vi "Handle Error.vi"(8 "error in (no error)":errorcluster, 11 "ModelLogsAndClearsErrors in":refnum<class "ModelLogsAndClearsErrors.lvclass">) -> (0 "error out":errorcluster, 2 "stop actor?":bool=TRUE, 3 "ModelLogsAndClearsErrors out":refnum<class "ModelLogsAndClearsErrors.lvclass">)   [LabVIEW 2020, in "ModelLogsAndClearsErrors.lvclass"]
doc: "(<B>Filename</B>: Actor Framework.lvlib:Actor.lvclass:Handle Error.vi)\n\nDefines how the actor handles an error that occurred while processing a message. By default, this method does nothing except stop the actor."
uses:
  ModelLogsAndClearsErrors.lvclass
  ModelLogsAndClearsErrors.lvclass/ModelLogsAndClearsErrors.ctl
  Source/IObserver/IObserver/IObserver.lvclass
  modules/composed-event-logger/Source/Composed Log/Types/Log Level.ctl
  modules/composed-event-logger/Source/Composed Log/Composed Log.lvlib
  ModelGeneratesError/ModelGeneratesError.lvclass
  C:/Git/mva-core/Test/Doubles/ModelGeneratesError/ModelGeneratesError.lvclass
  C:/Git/mva-core/Source/IModel/IModel/IModel.lvclass
  C:/Git/mva-core/Source/IObserver/IObserver/IObserver.lvclass
  C:/Program Files (x86)/National Instruments/LabVIEW 2020/vi.lib/ActorFramework/Actor/Actor.lvclass
  C:/Git/mva-core/Test/Doubles/ModelLogsAndClearsErrors/ModelLogsAndClearsErrors.lvclass
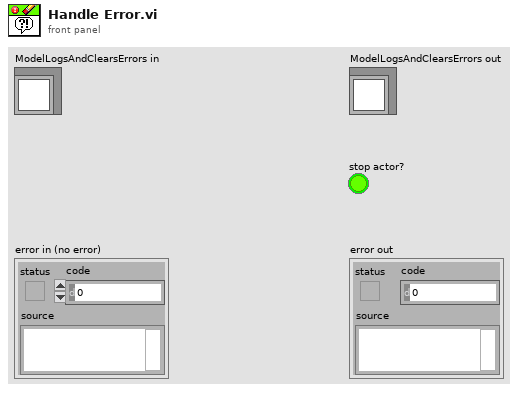
[diagram p1: front panel]
types:
  T1 = typedef "Composed Log.lvlib/Log Level.ctl" = enum16{"Debug", "Info", "Warning", "Error", "Critical"}
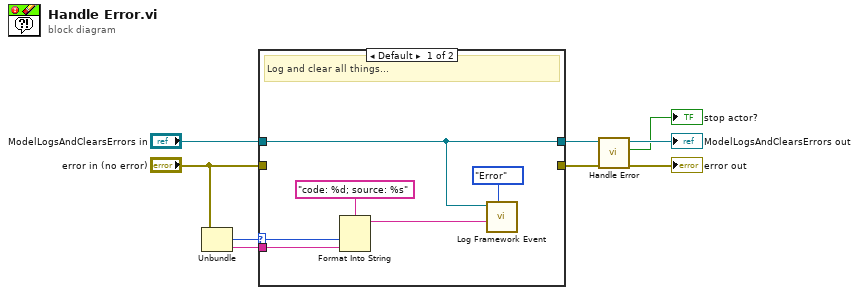
[diagram p0: block diagram]
diagram:
  n1 = Unbundle("error in (no error)") -> ("code"=w2:i32, "source"=w1:string)  [unwired: 1 out]
  n2 = case shown="Default" w2 {
    selector: w2 -> [w13 _]
    tunnel: "error in (no error)" -> [_ w16]
    tunnel: "ModelLogsAndClearsErrors in" -> [w15 w17]
    tunnel: [w15 w17] -> w5
    tunnel: [_ w16] -> w4
    tunnel: w1 -> [w12 _]
    frame Default {
      # "Log and clear all things..."
      n3 = Format Into String(format string="code: %d; source: %s", w13, w12) -> (resulting string=w10:string)  [unwired: 2 in, 1 out]
      n4 = call "Log Framework Event.vi"("Event Level (Debug)"=Log_Level."Error", "Data To Log"=w10, "IObserver in"=w15) -> ()  [unwired: 8 in, 1 out]
    }
    frame 43, 1608 {
      # "(that happens downstream)"
      # "...except stop codes"
    }
  }
  n5 = call-parent "Handle Error.vi"("error in (no error)"=w4, "IModel in"=w5) -> ("error out"=→"error out":errorcluster, "stop actor?"=→"stop actor?":bool, "IModel out"=→"ModelLogsAndClearsErrors out":refnum<class "ModelLogsAndClearsErrors.lvclass">)  [unwired: 7 in]
